vi "b.vi"() -> ()   [LabVIEW 2010]
uses:
  글로벌변수.vi
panel:
  out "a":dbl(graph)
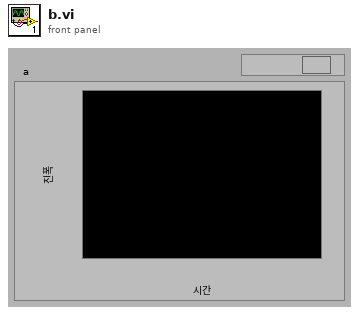
[diagram p1: front panel]
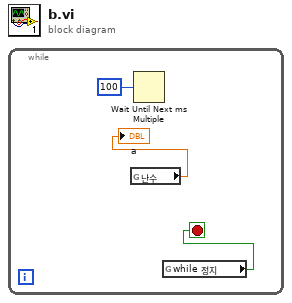
[diagram p0: block diagram]
diagram:
  n1 = while {
    stop <- w1 stop-if-true
    n2 = global read "글로벌변수.vi" "난수"() -> (→"a":dbl)
    n3 = Wait Until Next ms Multiple(millisecond multiple=u32 100 ("ms 배수")) -> ()  [unwired: 1 out]
    n4 = global read "글로벌변수.vi" "while 정지"() -> (w1:bool)
  }
